vi "Send Configure TV Trigger Line Number [TV].vi"(7 "Message Priority (Normal)":T1=enum."Normal", 8 "error in (no error)":errorcluster, 10 "tv line number (1)":i32=1, 11 "Message Enqueuer":refnum<class "Message Enqueuer.lvclass">) -> (0 "error out":errorcluster, 3 "Message Enqueuer out":refnum<class "Message Enqueuer.lvclass">)   [LabVIEW 2015, in "CS++Scope.lvlib" / "Configure TV Trigger Line Number [TV] Msg.lvclass"]
doc: "Sends the <B>CS++Scope.lvlib:Configure TV Trigger Line Number [TV] Msg.lvclass</B> message.\n\n<B>CS++Scope.lvlib:CS++Scope.lvclass:Configure TV Trigger Line Number [TV].vi</B> Description:\n\nThis VI configures the TV line upon which the oscilloscope triggers. The line number is absolute and not relative to the field of the TV signal.\n\nNote\n\n(1) This VI affects instrument behavior only if the trigger type is set to\n IVISCOPE_VAL_TV_TRIGGER and the TV trigger event is set to\n IVISCOPE_VAL_TV_EVENT_LINE_NUMBER. Call the IviScope\n Configure Trigger and the IviScope Configure TV Trigger Source [TV]\n VIs to set the trigger type and TV trigger event before calling this VI\n.\n(2) This VI is part of the IviScopeTVTrigger [TV] extension group."
uses:
  Configure TV Trigger Line Number [TV] Msg.lvclass
  <vilib>/ActorFramework/Message Enqueuer/Message Enqueuer.lvclass
  <vilib>/ActorFramework/Message Enqueuer/Message Priority.ctl
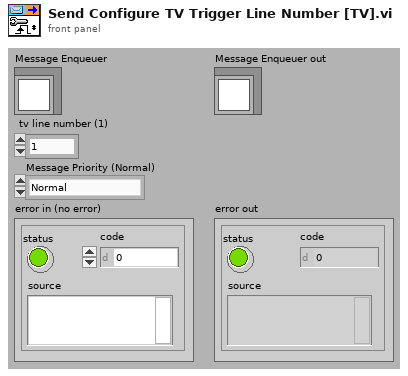
[diagram p1: front panel]
types:
  T1 = typedef "Actor Framework.lvlib/Message Enqueuer.lvclass/Message Priority.ctl" = enum16{"Low", "Normal", "High"}
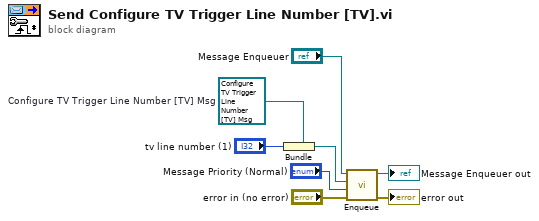
[diagram p0: block diagram]
diagram:
  w2 = refnum<class "Configure TV Trigger Line Number [TV] Msg.lvclass"> refnum  # Configure TV Trigger Line Number [TV] Msg
  n1 = Bundle(cluster=w2, "tv line number (1)") -> (w5:refnum<class "Configure TV Trigger Line Number [TV] Msg.lvclass">)
  n2 = call <vilib>:"Enqueue.vi"("error in (no error)"="error in (no error)", "Message Priority (Normal)"="Message Priority (Normal)", "Message"=w5, "Message Enqueuer in"="Message Enqueuer") -> ("error out"=→"error out":errorcluster, "Message Enqueuer out"=→"Message Enqueuer out":refnum<class "Message Enqueuer.lvclass">)  [unwired: 6 in]
